vi "RSNRPZ Set Scope Measurements Time.vi"(8 "error in (no error)":errorcluster, 9 "Meas Time (0.0)":dbl format="%^.3e", 10 "Channel (1)":i32=1, 11 "VISA session":refnum<visa-resource-name> caption="VISA resource name") -> (0 "error out":errorcluster, 3 "dup VISA session":refnum<visa-resource-name> caption="VISA resource name")   [LabVIEW 2010]
doc: "This VI defines measurement time which sets the duration of analysing the current trace for the pulse parameters. The measurement time could be used together with the measurement offset time to select the second (or any other) pulse in the trace and not the whole trace.\n\nNote:\n1) This VI is only available for NRP-Z81.\n\nRemote-control command(s):\nSENSe:TRACe:MEAS:TIME"
uses:
  rsnrpz_32.dll
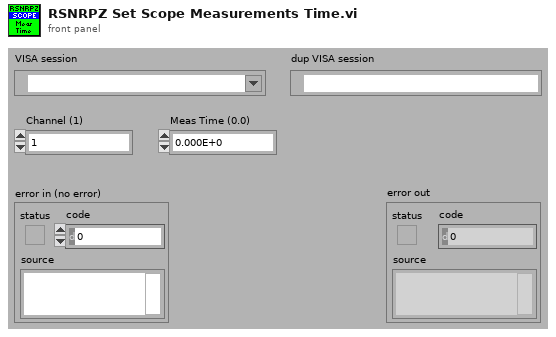
[diagram p1: front panel]
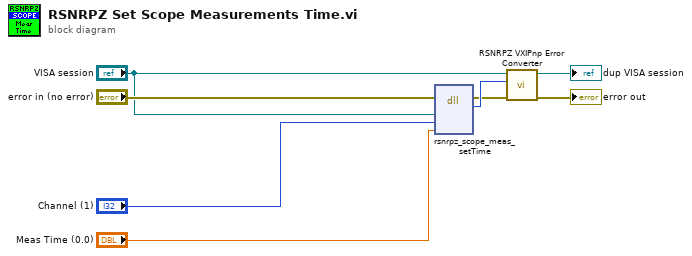
[diagram p0: block diagram]
diagram:
  n1 = dll-call lib="rsnrpz_32.dll" fn="rsnrpz_scope_meas_setTime"(error in="error in (no error)", "Instrument Handle"="VISA session", "Channel"="Channel (1)", "Meas Time"="Meas Time (0.0)") -> (error out=w5:errorcluster, w6:i32)  [unwired: 5 in, 1 out]
  n2 = call <instrlib>:"RSNRPZ VXIPnp Error Converter.vi"("error in"=w5, "VXIPnp error code"=w6, "VISA session"="VISA session") -> ("error out"=→"error out":errorcluster, "dup VISA session"=→"dup VISA session":refnum<visa-resource-name>)  [unwired: 7 in]
